vi "SendToExternalVariable.vi"(2 "error In":errorcluster, 3 "Igor Instruction String":string[](array[string]), 4 "Source of Data":refnum<k21>) -> (1 "error out":errorcluster)   [LabVIEW 2013]
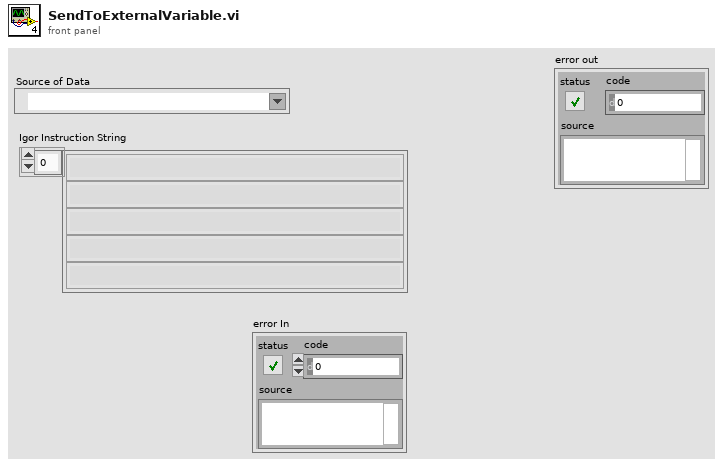
[diagram p1: front panel]
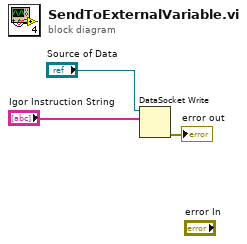
[diagram p0: block diagram]
diagram:
  n1 = DataSocket Write(10:"Igor Instruction String", 11:"Source of Data") -> (0:→"error out":errorcluster)  [unwired: 2 in, 2 out]
